vi "stop.vi"(8 "error in (no error)":errorcluster, 10 "stop?":bool, 11 "AtomChipHWC in":refnum<class "AtomChipHWC.lvclass">) -> (0 "error out":errorcluster, 2 "stopped":bool, 3 "AtomChipHWC out":refnum<class "AtomChipHWC.lvclass">)   [LabVIEW 2009, in "Hardware.lvlib" / "HWControllers.lvlib" / "AtomChipHWC.lvclass"]
doc: "Stop current run if input is true, otherwise ask hardware if its finished."
uses:
  AtomChipHWC.lvclass
  AtomChipHWC.lvclass/AtomChipHWC.ctl
  Channels/Digital/DigitalOutput.lvclass
  Channels/VoltOutput/AnalogOutput.lvclass
  Channels/DDSOutput/Generic/DDSOutput.lvclass
  Network Controllers/NetworkCamera/NetworkCamera.lvclass
  IntegrationManagement/CameraManager.lvclass
  HWController.lvclass
  Network Controllers/CameraNetworkController/CameraNetworkController.lvclass
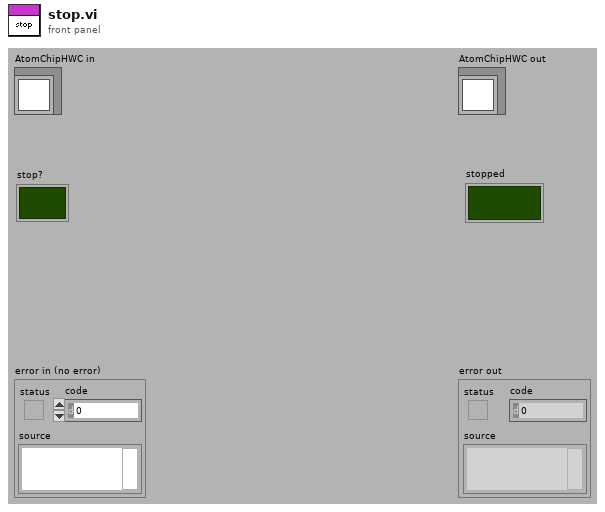
[diagram p1: front panel]
types:
  T1 = enum16{"Ready", "Compiling", "Configured", "Running", "Stopping", "Unresolved Error"}
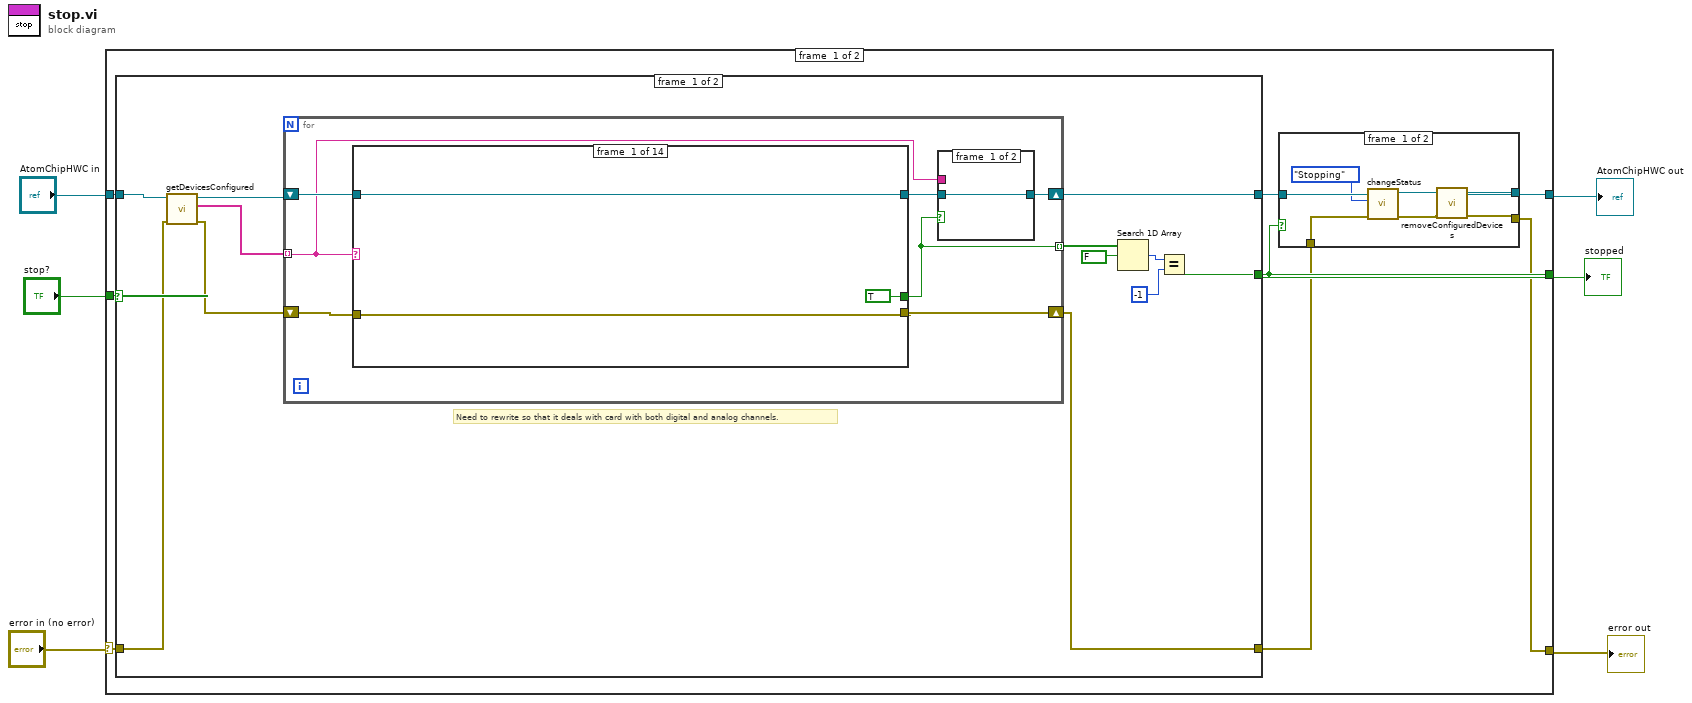
[diagram p0: block diagram]
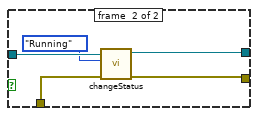
[diagram p2: hidden frame]
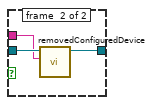
[diagram p3: hidden frame]
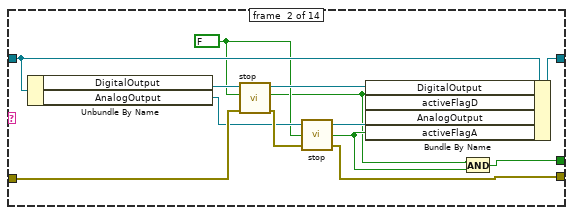
[diagram p4: hidden frame]
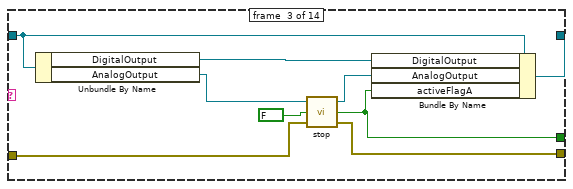
[diagram p5: hidden frame]
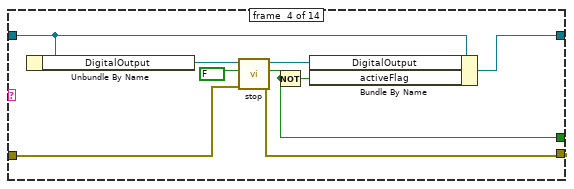
[diagram p6: hidden frame]
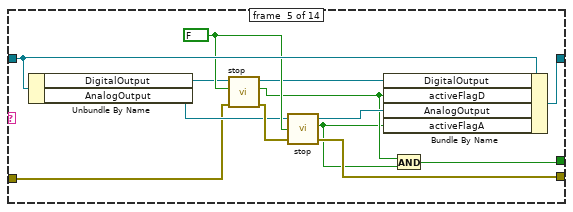
[diagram p7: hidden frame]
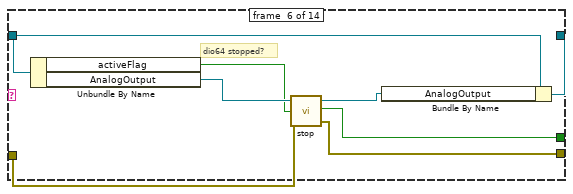
[diagram p8: hidden frame]
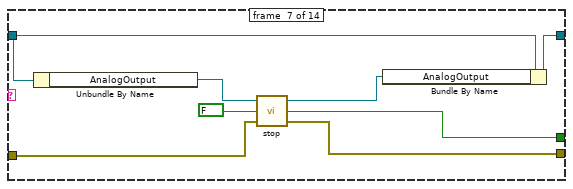
[diagram p9: hidden frame]
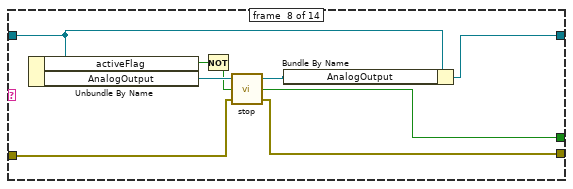
[diagram p10: hidden frame]
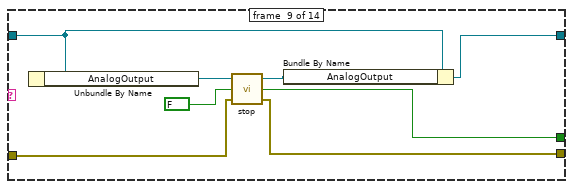
[diagram p11: hidden frame]
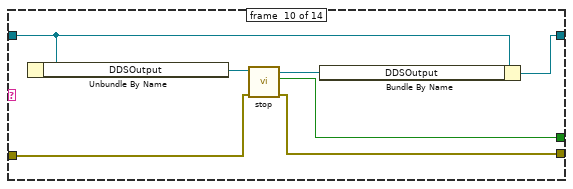
[diagram p12: hidden frame]
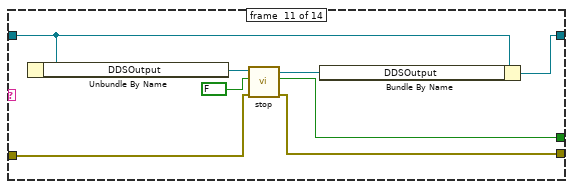
[diagram p13: hidden frame]
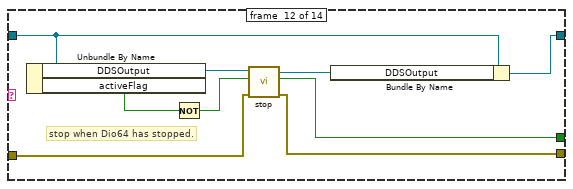
[diagram p14: hidden frame]
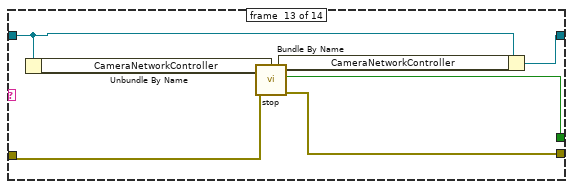
[diagram p15: hidden frame]
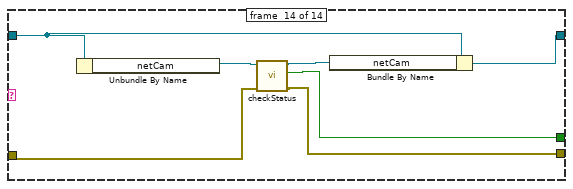
[diagram p16: hidden frame]
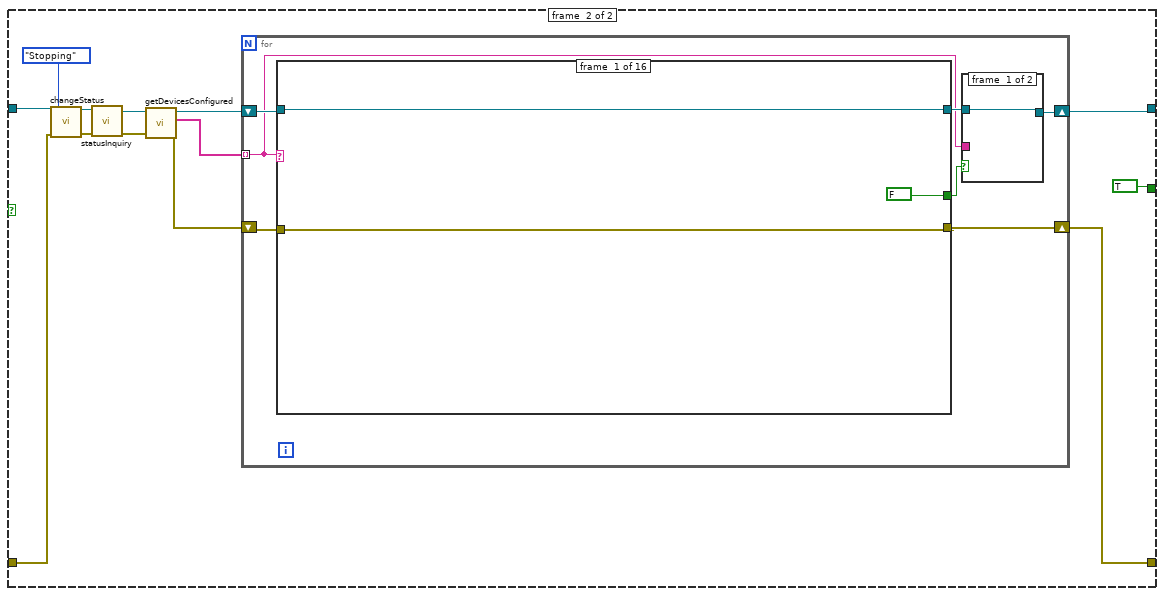
[diagram p17: hidden frame]
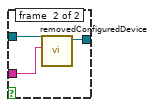
[diagram p18: hidden frame]
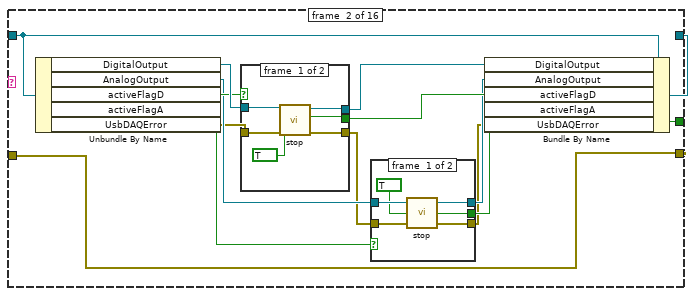
[diagram p19: hidden frame]
diagram:
  n1 = case shown="No Error" "error in (no error)" {
    selector: "error in (no error)" -> [w13 w375]
    tunnel: "AtomChipHWC in" -> [w14 w376]
    tunnel: [w8 w376] -> w5
    tunnel: [w7 w375] -> w3
    tunnel: "stop?" -> [w12 _]
    tunnel: [w9 _] -> w1
    frame #0 {
      n2 = case shown="False" w12 {
        tunnel: w14 -> [w31 w180]
        tunnel: [w38 w178] -> w11
        tunnel: w13 -> [w29 w179]
        tunnel: [w37 w177] -> w10
        tunnel: [w32 TRUE] -> w9
        frame #0 {
          # "Need to rewrite so that it deals with card with both digital and analog channels."
          n3 = call "getDevicesConfigured.vi"("error in (no error)"=w29, "HWController.lvclass in"=w31) -> ("error out"=w28:errorcluster, "devicesConfigured"=w27:string[], "HWController.lvclass out"=w30:refnum<class "AtomChipHWC.lvclass">)  [unwired: 7 in]
          n4 = for {
            shift-right: [w40] -> w38
            shift-left: w30 -> [w45]
            tunnel: w27 -> [w41] mode=indexing
            shift-right: [w44] -> w37
            shift-left: w28 -> [w43]
            tunnel: [w42] -> w36 mode=indexing
            n5 = case shown="\"Pixelfly\", \"ProEM_WinX32\"" w41 {
              tunnel: [w52 w64 w74 w79 w95 w104 w112 w115 w123 w130 w138 w147 w157 w166] -> w39
              tunnel: [w51 w61 w69 w81 w88 w101 w109 w119 w127 w134 w142 w151 w155 w162] -> w44
              tunnel: w45 -> [w52 w65 w72 w78 w96 w103 w111 w117 w125 w132 w140 w149 w158 w167]
              tunnel: w43 -> [w51 w59 w66 w82 w89 w99 w107 w120 w128 w135 w143 w152 w159 w163]
              tunnel: [TRUE w53 w67 w76 w84 w98 w105 w118 w126 w133 w141 w150 w156 w161] -> w42
              frame #0 {
              }
              frame #1 {
                w57 = FALSE
                n6 = Unbundle By Name(w65) -> ("DigitalOutput"=w63:refnum<class "DigitalOutput.lvclass">, "AnalogOutput"=w58:refnum<class "AnalogOutput.lvclass">)
                n7 = call-dynamic "stop.vi"("error in (no error)"=w59, "stop"=w57, "DigitalOutput in"=w63) -> ("error out"=w60:errorcluster, "stopped"=w54:bool, "DigitalOutput out"=w62:refnum<class "DigitalOutput.lvclass">)  [unwired: 6 in]
                n8 = call-dynamic "stop.vi"("error in (no error)"=w60, "stop"=w57, "AnalogOutput in"=w58) -> ("error out"=w61:errorcluster, "Stopped"=w55:bool, "AnalogOutput out"=w56:refnum<class "AnalogOutput.lvclass">)
                n9 = Bundle By Name(cluster=w65, "DigitalOutput"=w62, "activeFlagD"=w54, "AnalogOutput"=w56, "activeFlagA"=w55) -> (w64:refnum<class "AtomChipHWC.lvclass">)
                n10 = And(x=w54, y=w55) -> (x .and. y?=w53:bool)
              }
              frame #2 {
                n11 = Unbundle By Name(w72) -> ("DigitalOutput"=w68:refnum<class "DigitalOutput.lvclass">, "AnalogOutput"=w71:refnum<class "AnalogOutput.lvclass">)
                n12 = call-dynamic "stop.vi"("error in (no error)"=w66, "stop"=FALSE, "AnalogOutput in"=w71) -> ("error out"=w69:errorcluster, "Stopped"=w67:bool, "AnalogOutput out"=w70:refnum<class "AnalogOutput.lvclass">)
                n13 = Bundle By Name(cluster=w72, "DigitalOutput"=w68, "AnalogOutput"=w70, "activeFlagA"=w67) -> (w74:refnum<class "AtomChipHWC.lvclass">)
              }
              frame #3 {
                n14 = Unbundle By Name(w78) -> ("DigitalOutput"=w83:refnum<class "DigitalOutput.lvclass">)
                n15 = call-dynamic "stop.vi"("error in (no error)"=w82, "stop"=FALSE, "DigitalOutput in"=w83) -> ("error out"=w81:errorcluster, "stopped"=w76:bool, "DigitalOutput out"=w80:refnum<class "DigitalOutput.lvclass">)  [unwired: 6 in]
                n16 = Not(x=w76) -> (.not. x?=w75:bool)
                n17 = Bundle By Name(cluster=w78, "DigitalOutput"=w80, "activeFlag"=w75) -> (w79:refnum<class "AtomChipHWC.lvclass">)
              }
              frame #4 {
                w93 = FALSE
                n18 = Unbundle By Name(w96) -> ("DigitalOutput"=w92:refnum<class "DigitalOutput.lvclass">, "AnalogOutput"=w91:refnum<class "AnalogOutput.lvclass">)
                n19 = call-dynamic "stop.vi"("error in (no error)"=w89, "stop"=w93, "DigitalOutput in"=w92) -> ("error out"=w94:errorcluster, "stopped"=w86:bool, "DigitalOutput out"=w90:refnum<class "DigitalOutput.lvclass">)  [unwired: 6 in]
                n20 = call-dynamic "stop.vi"("error in (no error)"=w94, "stop"=w93, "AnalogOutput in"=w91) -> ("error out"=w88:errorcluster, "Stopped"=w85:bool, "AnalogOutput out"=w87:refnum<class "AnalogOutput.lvclass">)
                n21 = Bundle By Name(cluster=w96, "DigitalOutput"=w90, "activeFlagD"=w86, "AnalogOutput"=w87, "activeFlagA"=w85) -> (w95:refnum<class "AtomChipHWC.lvclass">)
                n22 = And(x=w86, y=w85) -> (x .and. y?=w84:bool)
              }
              frame #5 {
                # "dio64 stopped?"
                n23 = Unbundle By Name(w103) -> ("activeFlag"=w97:bool, "AnalogOutput"=w102:refnum<class "AnalogOutput.lvclass">)
                n24 = call-dynamic "stop.vi"("error in (no error)"=w99, "stop"=w97, "AnalogOutput in"=w102) -> ("error out"=w101:errorcluster, "Stopped"=w98:bool, "AnalogOutput out"=w100:refnum<class "AnalogOutput.lvclass">)
                n25 = Bundle By Name(cluster=w103, "AnalogOutput"=w100) -> (w104:refnum<class "AtomChipHWC.lvclass">)
              }
              frame #6 {
                n26 = Unbundle By Name(w111) -> ("AnalogOutput"=w110:refnum<class "AnalogOutput.lvclass">)
                n27 = call-dynamic "stop.vi"("error in (no error)"=w107, "stop"=FALSE, "AnalogOutput in"=w110) -> ("error out"=w109:errorcluster, "Stopped"=w105:bool, "AnalogOutput out"=w108:refnum<class "AnalogOutput.lvclass">)
                n28 = Bundle By Name(cluster=w111, "AnalogOutput"=w108) -> (w112:refnum<class "AtomChipHWC.lvclass">)
              }
              frame #7 {
                n29 = Unbundle By Name(w117) -> ("activeFlag"=w114:bool, "AnalogOutput"=w121:refnum<class "AnalogOutput.lvclass">)
                n30 = Not(x=w114) -> (.not. x?=w113:bool)
                n31 = call-dynamic "stop.vi"("error in (no error)"=w120, "stop"=w113, "AnalogOutput in"=w121) -> ("error out"=w119:errorcluster, "Stopped"=w118:bool, "AnalogOutput out"=w116:refnum<class "AnalogOutput.lvclass">)
                n32 = Bundle By Name(cluster=w117, "AnalogOutput"=w116) -> (w115:refnum<class "AtomChipHWC.lvclass">)
              }
              frame #8 {
                n33 = Unbundle By Name(w125) -> ("AnalogOutput"=w129:refnum<class "AnalogOutput.lvclass">)
                n34 = call-dynamic "stop.vi"("error in (no error)"=w128, "stop"=FALSE, "AnalogOutput in"=w129) -> ("error out"=w127:errorcluster, "Stopped"=w126:bool, "AnalogOutput out"=w124:refnum<class "AnalogOutput.lvclass">)
                n35 = Bundle By Name(cluster=w125, "AnalogOutput"=w124) -> (w123:refnum<class "AtomChipHWC.lvclass">)
              }
              frame #9 {
                n36 = Unbundle By Name(w132) -> ("DDSOutput"=w136:refnum<class "DDSOutput.lvclass">)
                n37 = call-dynamic "stop.vi"("error in (no error)"=w135, "DDSOutput in"=w136) -> ("error out"=w134:errorcluster, "hasStopped"=w133:bool, "DDSOutput out"=w131:refnum<class "DDSOutput.lvclass">)  [unwired: 7 in]
                n38 = Bundle By Name(cluster=w132, "DDSOutput"=w131) -> (w130:refnum<class "AtomChipHWC.lvclass">)
              }
              frame #10 {
                n39 = Unbundle By Name(w140) -> ("DDSOutput"=w144:refnum<class "DDSOutput.lvclass">)
                n40 = call-dynamic "stop.vi"("error in (no error)"=w143, "stop?"=FALSE, "DDSOutput in"=w144) -> ("error out"=w142:errorcluster, "hasStopped"=w141:bool, "DDSOutput out"=w139:refnum<class "DDSOutput.lvclass">)  [unwired: 6 in]
                n41 = Bundle By Name(cluster=w140, "DDSOutput"=w139) -> (w138:refnum<class "AtomChipHWC.lvclass">)
              }
              frame #11 {
                # "stop when Dio64 has stopped."
                n42 = Unbundle By Name(w149) -> ("DDSOutput"=w153:refnum<class "DDSOutput.lvclass">, "activeFlag"=w146:bool)
                n43 = Not(x=w146) -> (.not. x?=w145:bool)
                n44 = call-dynamic "stop.vi"("error in (no error)"=w152, "stop?"=w145, "DDSOutput in"=w153) -> ("error out"=w151:errorcluster, "hasStopped"=w150:bool, "DDSOutput out"=w148:refnum<class "DDSOutput.lvclass">)  [unwired: 6 in]
                n45 = Bundle By Name(cluster=w149, "DDSOutput"=w148) -> (w147:refnum<class "AtomChipHWC.lvclass">)
              }
              frame #12 {
                n46 = Unbundle By Name(w158) -> ("CameraNetworkController"=w160:refnum<class "CameraNetworkController.lvclass">)
                n47 = call "stop.vi"("error in (no error)"=w159, "CameraNetworkController in"=w160) -> ("error out"=w155:errorcluster, "stopped?"=w156:bool, "CameraNetworkController out"=w154:refnum<class "CameraNetworkController.lvclass">)  [unwired: 7 in]
                n48 = Bundle By Name(cluster=w158, "CameraNetworkController"=w154) -> (w157:refnum<class "AtomChipHWC.lvclass">)
              }
              frame #13 {
                n49 = Unbundle By Name(w167) -> ("netCam"=w165:refnum<class "NetworkCamera.lvclass">)
                n50 = call-dynamic "checkStatus.vi"("error in (no error)"=w163, "NetworkCamera in"=w165) -> ("error out"=w162:errorcluster, "stopped?"=w161:bool, "NetworkCamera out"=w164:refnum<class "NetworkCamera.lvclass">)  [unwired: 7 in]
                n51 = Bundle By Name(cluster=w167, "netCam"=w164) -> (w166:refnum<class "AtomChipHWC.lvclass">)
              }
            }
            n52 = case shown="True" w42 {
              tunnel: w41 -> [_ w47]
              tunnel: [w46 w48] -> w40
              tunnel: w39 -> [w46 w49]
              frame #0 {
              }
              frame #1 {
                n53 = call-dynamic "removedConfiguredDevice.vi"("device"=w47, "HWController in"=w49) -> ("HWController out"=w48:refnum<class "AtomChipHWC.lvclass">)  [unwired: 8 in, 1 out]
              }
            }
          }
          n54 = Search 1D Array(1D array=w36, element=FALSE) -> (index of element=w34:i32)  [unwired: 1 in]
          n55 = Equal?(x=w34, y=-1) -> (x = y?=w32:bool)
        }
        frame #1 {
          n56 = call "changeStatus.vi"("error in (no error)"=w179, "status"=T1."Stopping", "HWController in"=w180) -> ("error out"=w174:errorcluster, "HWController out"=w175:refnum<class "AtomChipHWC.lvclass">)  [unwired: 7 in]
          n57 = call-dynamic "statusInquiry.vi"("error in (no error)"=w174, "HWController in"=w175) -> ("error out"=w170:errorcluster, "HWController out"=w173:refnum<class "AtomChipHWC.lvclass">)  [unwired: 8 in]
          n58 = call "getDevicesConfigured.vi"("error in (no error)"=w170, "HWController.lvclass in"=w173) -> ("error out"=w169:errorcluster, "devicesConfigured"=w171:string[], "HWController.lvclass out"=w172:refnum<class "AtomChipHWC.lvclass">)  [unwired: 7 in]
          n59 = for {
            tunnel: w171 -> [w182] mode=indexing
            shift-right: [w183] -> w178
            shift-left: w172 -> [w187]
            shift-right: [w185] -> w177
            shift-left: w169 -> [w186]
            n60 = case shown="\"Pixelfly\", \"ProEM_WinX32\"" w182 {
              tunnel: [w194 w201 w234 w242 w259 w286 w292 w300 w308 w316 w325 w336 w345 w354 w364 w373] -> w184
              tunnel: [w193 w195 w227 w237 w246 w278 w287 w298 w304 w312 w321 w330 w339 w348 w359 w372] -> w185
              tunnel: w187 -> [w194 w200 w233 w243 w258 w285 w293 w302 w310 w317 w326 w337 w346 w355 w365 w374]
              tunnel: w186 -> [w193 w195 w227 w237 w246 w278 w287 w298 w304 w312 w321 w330 w339 w348 w359 w372]
              tunnel: [FALSE w199 w230 w241 w251 w281 w291 TRUE TRUE w315 w324 w334 w343 w352 w360 w366] -> w181
              frame #0 {
              }
              frame #1 {
                n61 = Unbundle By Name(w200) -> ("DigitalOutput"=w208:refnum<class "DigitalOutput.lvclass">, "AnalogOutput"=w205:refnum<class "AnalogOutput.lvclass">, "activeFlagD"=w207:bool, "activeFlagA"=w204:bool, "UsbDAQError"=w196:errorcluster)
                n62 = case shown="False" w207 {
                  selector: w207 -> [_ w224]
                  tunnel: w208 -> [w223 w226]
                  tunnel: [w222 w226] -> w206
                  tunnel: w196 -> [w221 w225]
                  tunnel: [w220 w225] -> w198
                  tunnel: [w218 w224] -> w203
                  frame #0 {
                    n63 = call-dynamic "stop.vi"("error in (no error)"=w221, "stop"=TRUE, "DigitalOutput in"=w223) -> ("error out"=w220:errorcluster, "stopped"=w218:bool, "DigitalOutput out"=w222:refnum<class "DigitalOutput.lvclass">)  [unwired: 6 in]
                  }
                  frame #1 {
                  }
                }
                n64 = case shown="False" w204 {
                  selector: w204 -> [_ w215]
                  tunnel: w198 -> [w214 w216]
                  tunnel: w205 -> [w213 w217]
                  tunnel: [w211 w217] -> w202
                  tunnel: [w210 w216] -> w197
                  tunnel: [w209 w215] -> w199
                  frame #0 {
                    n65 = call-dynamic "stop.vi"("error in (no error)"=w214, "stop"=TRUE, "AnalogOutput in"=w213) -> ("error out"=w210:errorcluster, "Stopped"=w209:bool, "AnalogOutput out"=w211:refnum<class "AnalogOutput.lvclass">)
                  }
                  frame #1 {
                  }
                }
                n66 = Bundle By Name(cluster=w200, "DigitalOutput"=w206, "AnalogOutput"=w202, "activeFlagD"=w203, "activeFlagA"=w199, "UsbDAQError"=w197) -> (w201:refnum<class "AtomChipHWC.lvclass">)
              }
              frame #2 {
                n67 = Unbundle By Name(w233) -> ("DigitalOutput"=w232:refnum<class "DigitalOutput.lvclass">, "AnalogOutput"=w236:refnum<class "AnalogOutput.lvclass">, "daqError"=w228:errorcluster)
                n68 = call-dynamic "stop.vi"("error in (no error)"=w228, "stop"=TRUE, "AnalogOutput in"=w236) -> ("error out"=w229:errorcluster, "Stopped"=w230:bool, "AnalogOutput out"=w235:refnum<class "AnalogOutput.lvclass">)
                n69 = Bundle By Name(cluster=w233, "DigitalOutput"=w232, "AnalogOutput"=w235, "activeFlagA"=w230, "daqError"=w229) -> (w234:refnum<class "AtomChipHWC.lvclass">)
              }
              frame #3 {
                n70 = Unbundle By Name(w243) -> ("DigitalOutput"=w245:refnum<class "DigitalOutput.lvclass">, "Dio64Error"=w238:errorcluster)
                n71 = call-dynamic "stop.vi"("error in (no error)"=w238, "stop"=TRUE, "DigitalOutput in"=w245) -> ("error out"=w239:errorcluster, "stopped"=w241:bool, "DigitalOutput out"=w244:refnum<class "DigitalOutput.lvclass">)  [unwired: 6 in]
                n72 = Bundle By Name(cluster=w243, "DigitalOutput"=w244, "activeFlag"=w241, "Dio64Error"=w239) -> (w242:refnum<class "AtomChipHWC.lvclass">)
              }
              frame #4 {
                n73 = Unbundle By Name(w258) -> ("DigitalOutput"=w257:refnum<class "DigitalOutput.lvclass">, "AnalogOutput"=w248:refnum<class "AnalogOutput.lvclass">, "activeFlagD"=w256:bool, "activeFlagA"=w250:bool, "Ao8Error"=w247:errorcluster)
                n74 = case shown="False" w256 {
                  selector: w256 -> [_ w275]
                  tunnel: w257 -> [w274 w277]
                  tunnel: [w273 w277] -> w255
                  tunnel: w247 -> [w272 w276]
                  tunnel: [w271 w276] -> w254
                  tunnel: [w269 w275] -> w253
                  frame #0 {
                    n75 = call-dynamic "stop.vi"("error in (no error)"=w272, "stop"=TRUE, "DigitalOutput in"=w274) -> ("error out"=w271:errorcluster, "stopped"=w269:bool, "DigitalOutput out"=w273:refnum<class "DigitalOutput.lvclass">)  [unwired: 6 in]
                  }
                  frame #1 {
                  }
                }
                n76 = case shown="False" w250 {
                  selector: w250 -> [_ w266]
                  tunnel: w254 -> [w265 w267]
                  tunnel: w248 -> [w264 w268]
                  tunnel: [w262 w268] -> w252
                  tunnel: [w261 w267] -> w249
                  tunnel: [w260 w266] -> w251
                  frame #0 {
                    n77 = call-dynamic "stop.vi"("error in (no error)"=w265, "stop"=TRUE, "AnalogOutput in"=w264) -> ("error out"=w261:errorcluster, "Stopped"=w260:bool, "AnalogOutput out"=w262:refnum<class "AnalogOutput.lvclass">)
                  }
                  frame #1 {
                  }
                }
                n78 = Bundle By Name(cluster=w258, "DigitalOutput"=w255, "AnalogOutput"=w252, "activeFlagD"=w253, "activeFlagA"=w251, "Ao8Error"=w249) -> (w259:refnum<class "AtomChipHWC.lvclass">)
              }
              frame #5 {
                n79 = Unbundle By Name(w285) -> ("AnalogOutput"=w284:refnum<class "AnalogOutput.lvclass">, "Ao32Error"=w280:errorcluster)
                n80 = call-dynamic "stop.vi"("error in (no error)"=w280, "stop"=TRUE, "AnalogOutput in"=w284) -> ("error out"=w279:errorcluster, "Stopped"=w281:bool, "AnalogOutput out"=w283:refnum<class "AnalogOutput.lvclass">)
                n81 = Bundle By Name(cluster=w285, "AnalogOutput"=w283, "Ao32Error"=w279) -> (w286:refnum<class "AtomChipHWC.lvclass">)
              }
              frame #6 {
                n82 = Unbundle By Name(w293) -> ("AnalogOutput"=w295:refnum<class "AnalogOutput.lvclass">, "daqError"=w289:errorcluster)
                n83 = call-dynamic "stop.vi"("error in (no error)"=w289, "stop"=TRUE, "AnalogOutput in"=w295) -> ("error out"=w288:errorcluster, "Stopped"=w291:bool, "AnalogOutput out"=w294:refnum<class "AnalogOutput.lvclass">)
                n84 = Bundle By Name(cluster=w293, "AnalogOutput"=w294, "daqError"=w288) -> (w292:refnum<class "AtomChipHWC.lvclass">)
              }
              frame #7 {
                n85 = Unbundle By Name(w302) -> ("CameraManager"=w303:refnum<class "CameraManager.lvclass">, "ICCameraError"=w297:errorcluster)
                n86 = call-dynamic "stopSnapping.vi"("error in (no error)"=w297, "CameraManager in"=w303) -> ("error out"=w296:errorcluster, "CameraManager out"=w301:refnum<class "CameraManager.lvclass">)  [unwired: 8 in]
                n87 = Bundle By Name(cluster=w302, "CameraManager"=w301, "ICCameraError"=w296) -> (w300:refnum<class "AtomChipHWC.lvclass">)
              }
              frame #8 {
                n88 = Unbundle By Name(w310) -> ("CameraManager"=w311:refnum<class "CameraManager.lvclass">, "AndorIkonError"=w306:errorcluster)
                n89 = call-dynamic "stopSnapping.vi"("error in (no error)"=w306, "CameraManager in"=w311) -> ("error out"=w305:errorcluster, "CameraManager out"=w309:refnum<class "CameraManager.lvclass">)  [unwired: 8 in]
                n90 = Bundle By Name(cluster=w310, "CameraManager"=w309, "AndorIkonError"=w305) -> (w308:refnum<class "AtomChipHWC.lvclass">)
              }
              frame #9 {
                n91 = Unbundle By Name(w317) -> ("AnalogOutput"=w319:refnum<class "AnalogOutput.lvclass">, "Ao8aError"=w314:errorcluster)
                n92 = call-dynamic "stop.vi"("error in (no error)"=w314, "stop"=TRUE, "AnalogOutput in"=w319) -> ("error out"=w313:errorcluster, "Stopped"=w315:bool, "AnalogOutput out"=w318:refnum<class "AnalogOutput.lvclass">)
                n93 = Bundle By Name(cluster=w317, "AnalogOutput"=w318, "Ao8aError"=w313) -> (w316:refnum<class "AtomChipHWC.lvclass">)
              }
              frame #10 {
                n94 = Unbundle By Name(w326) -> ("AnalogOutput"=w328:refnum<class "AnalogOutput.lvclass">, "Ao8bError"=w323:errorcluster)
                n95 = call-dynamic "stop.vi"("error in (no error)"=w323, "stop"=TRUE, "AnalogOutput in"=w328) -> ("error out"=w322:errorcluster, "Stopped"=w324:bool, "AnalogOutput out"=w327:refnum<class "AnalogOutput.lvclass">)
                n96 = Bundle By Name(cluster=w326, "AnalogOutput"=w327, "Ao8bError"=w322) -> (w325:refnum<class "AtomChipHWC.lvclass">)
              }
              frame #11 {
                n97 = Unbundle By Name(w337) -> ("DDSOutput"=w338:refnum<class "DDSOutput.lvclass">, "DDS0Error"=w332:errorcluster)
                n98 = call-dynamic "stop.vi"("error in (no error)"=w332, "stop?"=TRUE, "DDSOutput in"=w338) -> ("error out"=w331:errorcluster, "hasStopped"=w334:bool, "DDSOutput out"=w335:refnum<class "DDSOutput.lvclass">)  [unwired: 6 in]
                n99 = Bundle By Name(cluster=w337, "DDSOutput"=w335, "DDS0Error"=w331) -> (w336:refnum<class "AtomChipHWC.lvclass">)
              }
              frame #12 {
                n100 = Unbundle By Name(w346) -> ("DDSOutput"=w347:refnum<class "DDSOutput.lvclass">, "DDS1Error"=w340:errorcluster)
                n101 = call-dynamic "stop.vi"("error in (no error)"=w340, "stop?"=TRUE, "DDSOutput in"=w347) -> ("error out"=w341:errorcluster, "hasStopped"=w343:bool, "DDSOutput out"=w344:refnum<class "DDSOutput.lvclass">)  [unwired: 6 in]
                n102 = Bundle By Name(cluster=w346, "DDSOutput"=w344, "DDS1Error"=w341) -> (w345:refnum<class "AtomChipHWC.lvclass">)
              }
              frame #13 {
                n103 = Unbundle By Name(w355) -> ("DDSOutput"=w356:refnum<class "DDSOutput.lvclass">, "DDS0Error"=w349:errorcluster)
                n104 = call-dynamic "stop.vi"("error in (no error)"=w349, "stop?"=TRUE, "DDSOutput in"=w356) -> ("error out"=w350:errorcluster, "hasStopped"=w352:bool, "DDSOutput out"=w353:refnum<class "DDSOutput.lvclass">)  [unwired: 6 in]
                n105 = Bundle By Name(cluster=w355, "DDSOutput"=w353, "DDS0Error"=w350) -> (w354:refnum<class "AtomChipHWC.lvclass">)
              }
              frame #14 {
                n106 = Unbundle By Name(w365) -> ("CameraNetworkController"=w363:refnum<class "CameraNetworkController.lvclass">, "CameraNError"=w358:errorcluster)
                n107 = call "stop.vi"("error in (no error)"=w358, "stop"=TRUE, "CameraNetworkController in"=w363) -> ("error out"=w357:errorcluster, "stopped?"=w360:bool, "CameraNetworkController out"=w362:refnum<class "CameraNetworkController.lvclass">)  [unwired: 6 in]
                n108 = Bundle By Name(cluster=w365, "CameraNetworkController"=w362, "CameraNError"=w357) -> (w364:refnum<class "AtomChipHWC.lvclass">)
              }
              frame #15 {
                n109 = Unbundle By Name(w374) -> ("netCam"=w370:refnum<class "NetworkCamera.lvclass">, "netCamError"=w369:errorcluster)
                n110 = call-dynamic "checkStatus.vi"("error in (no error)"=w369, "stop"=TRUE, "NetworkCamera in"=w370) -> ("error out"=w368:errorcluster, "stopped?"=w366:bool, "NetworkCamera out"=w371:refnum<class "NetworkCamera.lvclass">)  [unwired: 6 in]
                n111 = Bundle By Name(cluster=w374, "netCam"=w371, "netCamError"=w368) -> (w373:refnum<class "AtomChipHWC.lvclass">)
              }
            }
            n112 = case shown="True" w181 {
              tunnel: w184 -> [w188 w191]
              tunnel: [w188 w190] -> w183
              tunnel: w182 -> [_ w189]
              frame #0 {
              }
              frame #1 {
                n113 = call-dynamic "removedConfiguredDevice.vi"("device"=w189, "HWController in"=w191) -> ("HWController out"=w190:refnum<class "AtomChipHWC.lvclass">)  [unwired: 8 in, 1 out]
              }
            }
          }
        }
      }
      n114 = case shown="True" w9 {
        tunnel: w11 -> [w21 w26]
        tunnel: [w15 w25] -> w8
        tunnel: w10 -> [w20 w24]
        tunnel: [w16 w23] -> w7
        frame #0 {
          n115 = call "changeStatus.vi"("error in (no error)"=w20, "status"=T1."Stopping", "HWController in"=w21) -> ("error out"=w17:errorcluster, "HWController out"=w18:refnum<class "AtomChipHWC.lvclass">)  [unwired: 7 in]
          n116 = call "removeConfiguredDevices.vi"("error in (no error)"=w17, "HWController in"=w18) -> ("error out"=w16:errorcluster, "HWController out"=w15:refnum<class "AtomChipHWC.lvclass">)  [unwired: 8 in]
        }
        frame #1 {
          n117 = call "changeStatus.vi"("error in (no error)"=w24, "status"=T1."Running", "HWController in"=w26) -> ("error out"=w23:errorcluster, "HWController out"=w25:refnum<class "AtomChipHWC.lvclass">)  [unwired: 7 in]
        }
      }
    }
    frame #1 {
    }
  }
  "error out" <- w3
  "AtomChipHWC out" <- w5
  "stopped" <- w1
